vi "Inficon 32 Bit Data.vi"(6 "HHV Manual Mode?":bool, 7 "Gas Type":enum16{"Natural Gas", "Propane Gas"}(ring), 8 "Error In":errorcluster, 9 "Gross Heating Value (Dry) - Manual":sgl, 10 "Inficon Data Input":T3={"Gross Heating Value, Vol (Real, Dry)"=65535.0, "Nitrogen Component Normalized Mole % (Dry)"=8.0, "Methane Component Normalized Mole % (Dry)"=69.0, "Carbon Dioxide Component Normalized Mole % (Dry)"=65535.0, "Ethane Component Normalized Mole % (Dry)"=65.0, "Propane Component Normalized Mole % (Dry)"=8.0, "i-Pentane Component Normalized Mole % (Dry)"=14.0, "i-Butane Component Normalized Mole % (Dry)"=66.0, "n-Butane Component Normalized Mole % (Dry)"=8.0, "n-Pentane Component Normalized Mole % (Dry)"=0.0, "Hexane Component Normalized Mole % (Dry)"=0.0, "Heptane Component Normalized Mole % (Dry)"=0.0, "Gross Wobbe Index, Real(Dry)"=0.0, "Relative Density, Real(Dry)"=40.0, "Propylene Component Normalized Mole % (Dry)"=0.0, "C4 Olefins Component Normalized Mole % (Dry)"=0.0, "Water Component Normalized Mole % (Dry)"=0.0}, 11 "Modbus master in":refnum<class "Modbus Master.lvclass">=refnum) -> (0 "Error Out":errorcluster, 2 "Inficon Data Output":T3, 3 "Modbus master out":refnum<class "Modbus Master.lvclass">, 5 "Text Array":string[][](array[string]))   [LabVIEW 2020]
uses:
  Type Definitions/Inficon Data.ctl
  <vilib>/NI/Modbus Library/API/Master/Modbus Master.lvclass
  <vilib>/NI/Modbus Library/Transmission Data Unit/IP/IP Data Unit.lvclass
  <vilib>/NI/Modbus Library/Master Function Definition/Master Function Definition.lvclass
  <vilib>/NI/Modbus Library/Network Protocol/Network Master/TCP/TCP Master.lvclass
  Type Definitions/Inficon Modbus Addresses.ctl
  Type Definitions/Inficon Modbus Addresses LP.ctl
panel:
  in  "Density LP":T1=126 items=["Gross Heating Value (Dry)"=100, "Ethane"=102, "Propane"=104, "Proplyene"=106, "i-Butane"=108, "n-butane"=110, "C4 Olefins"=112, "Water"=114, "Gross Wobbe Index (Dry)"=124, "Relative Density (Dry)"=126]
  in  "Wobbe LP":T1=124 items=["Gross Heating Value (Dry)"=100, "Ethane"=102, "Propane"=104, "Proplyene"=106, "i-Butane"=108, "n-butane"=110, "C4 Olefins"=112, "Water"=114, "Gross Wobbe Index (Dry)"=124, "Relative Density (Dry)"=126]
  in  "Water":T1=114 items=["Gross Heating Value (Dry)"=100, "Ethane"=102, "Propane"=104, "Proplyene"=106, "i-Butane"=108, "n-butane"=110, "C4 Olefins"=112, "Water"=114, "Gross Wobbe Index (Dry)"=124, "Relative Density (Dry)"=126]
  in  "C4":T1=112 items=["Gross Heating Value (Dry)"=100, "Ethane"=102, "Propane"=104, "Proplyene"=106, "i-Butane"=108, "n-butane"=110, "C4 Olefins"=112, "Water"=114, "Gross Wobbe Index (Dry)"=124, "Relative Density (Dry)"=126]
  in  "n-Butane LP":T1=110 items=["Gross Heating Value (Dry)"=100, "Ethane"=102, "Propane"=104, "Proplyene"=106, "i-Butane"=108, "n-butane"=110, "C4 Olefins"=112, "Water"=114, "Gross Wobbe Index (Dry)"=124, "Relative Density (Dry)"=126]
  in  "i-Butane LP":T1=108 items=["Gross Heating Value (Dry)"=100, "Ethane"=102, "Propane"=104, "Proplyene"=106, "i-Butane"=108, "n-butane"=110, "C4 Olefins"=112, "Water"=114, "Gross Wobbe Index (Dry)"=124, "Relative Density (Dry)"=126]
  in  "Proplyene":T1=106 items=["Gross Heating Value (Dry)"=100, "Ethane"=102, "Propane"=104, "Proplyene"=106, "i-Butane"=108, "n-butane"=110, "C4 Olefins"=112, "Water"=114, "Gross Wobbe Index (Dry)"=124, "Relative Density (Dry)"=126]
  in  "Propane":T1=104 items=["Gross Heating Value (Dry)"=100, "Ethane"=102, "Propane"=104, "Proplyene"=106, "i-Butane"=108, "n-butane"=110, "C4 Olefins"=112, "Water"=114, "Gross Wobbe Index (Dry)"=124, "Relative Density (Dry)"=126]
  in  "Ethane":T1=102 items=["Gross Heating Value (Dry)"=100, "Ethane"=102, "Propane"=104, "Proplyene"=106, "i-Butane"=108, "n-butane"=110, "C4 Olefins"=112, "Water"=114, "Gross Wobbe Index (Dry)"=124, "Relative Density (Dry)"=126]
  in  "HHV LP":T1=100 items=["Gross Heating Value (Dry)"=100, "Ethane"=102, "Propane"=104, "Proplyene"=106, "i-Butane"=108, "n-butane"=110, "C4 Olefins"=112, "Water"=114, "Gross Wobbe Index (Dry)"=124, "Relative Density (Dry)"=126]
  in  "Density NG":T2=126 items=["Gross Heating Value (Dry)"=100, "Nitrogen"=102, "Methane"=104, "CO2"=106, "Ethane"=108, "Propane"=110, "i-Butane"=112, "n-Butane"=114, "i-Pentane"=116, "n-Pentane"=118, "Hexane"=120, "Heptane"=122, "Gross Wobbe Index (Dry)"=124, "Relative Density (Dry)"=126]
  in  "Wobbe NG":T2=124 items=["Gross Heating Value (Dry)"=100, "Nitrogen"=102, "Methane"=104, "CO2"=106, "Ethane"=108, "Propane"=110, "i-Butane"=112, "n-Butane"=114, "i-Pentane"=116, "n-Pentane"=118, "Hexane"=120, "Heptane"=122, "Gross Wobbe Index (Dry)"=124, "Relative Density (Dry)"=126]
  in  "Heptane":T2=122 items=["Gross Heating Value (Dry)"=100, "Nitrogen"=102, "Methane"=104, "CO2"=106, "Ethane"=108, "Propane"=110, "i-Butane"=112, "n-Butane"=114, "i-Pentane"=116, "n-Pentane"=118, "Hexane"=120, "Heptane"=122, "Gross Wobbe Index (Dry)"=124, "Relative Density (Dry)"=126]
  in  "Hexane":T2=120 items=["Gross Heating Value (Dry)"=100, "Nitrogen"=102, "Methane"=104, "CO2"=106, "Ethane"=108, "Propane"=110, "i-Butane"=112, "n-Butane"=114, "i-Pentane"=116, "n-Pentane"=118, "Hexane"=120, "Heptane"=122, "Gross Wobbe Index (Dry)"=124, "Relative Density (Dry)"=126]
  in  "n-Pentane":T2=118 items=["Gross Heating Value (Dry)"=100, "Nitrogen"=102, "Methane"=104, "CO2"=106, "Ethane"=108, "Propane"=110, "i-Butane"=112, "n-Butane"=114, "i-Pentane"=116, "n-Pentane"=118, "Hexane"=120, "Heptane"=122, "Gross Wobbe Index (Dry)"=124, "Relative Density (Dry)"=126]
  in  "i-Pentane":T2=116 items=["Gross Heating Value (Dry)"=100, "Nitrogen"=102, "Methane"=104, "CO2"=106, "Ethane"=108, "Propane"=110, "i-Butane"=112, "n-Butane"=114, "i-Pentane"=116, "n-Pentane"=118, "Hexane"=120, "Heptane"=122, "Gross Wobbe Index (Dry)"=124, "Relative Density (Dry)"=126]
  in  "n-Butane":T2=114 items=["Gross Heating Value (Dry)"=100, "Nitrogen"=102, "Methane"=104, "CO2"=106, "Ethane"=108, "Propane"=110, "i-Butane"=112, "n-Butane"=114, "i-Pentane"=116, "n-Pentane"=118, "Hexane"=120, "Heptane"=122, "Gross Wobbe Index (Dry)"=124, "Relative Density (Dry)"=126]
  in  "i-Butane":T2=112 items=["Gross Heating Value (Dry)"=100, "Nitrogen"=102, "Methane"=104, "CO2"=106, "Ethane"=108, "Propane"=110, "i-Butane"=112, "n-Butane"=114, "i-Pentane"=116, "n-Pentane"=118, "Hexane"=120, "Heptane"=122, "Gross Wobbe Index (Dry)"=124, "Relative Density (Dry)"=126]
  in  "Propane":T2=110 items=["Gross Heating Value (Dry)"=100, "Nitrogen"=102, "Methane"=104, "CO2"=106, "Ethane"=108, "Propane"=110, "i-Butane"=112, "n-Butane"=114, "i-Pentane"=116, "n-Pentane"=118, "Hexane"=120, "Heptane"=122, "Gross Wobbe Index (Dry)"=124, "Relative Density (Dry)"=126]
  in  "Ethane":T2=108 items=["Gross Heating Value (Dry)"=100, "Nitrogen"=102, "Methane"=104, "CO2"=106, "Ethane"=108, "Propane"=110, "i-Butane"=112, "n-Butane"=114, "i-Pentane"=116, "n-Pentane"=118, "Hexane"=120, "Heptane"=122, "Gross Wobbe Index (Dry)"=124, "Relative Density (Dry)"=126]
  in  "CO2":T2=106 items=["Gross Heating Value (Dry)"=100, "Nitrogen"=102, "Methane"=104, "CO2"=106, "Ethane"=108, "Propane"=110, "i-Butane"=112, "n-Butane"=114, "i-Pentane"=116, "n-Pentane"=118, "Hexane"=120, "Heptane"=122, "Gross Wobbe Index (Dry)"=124, "Relative Density (Dry)"=126]
  in  "CH4":T2=104 items=["Gross Heating Value (Dry)"=100, "Nitrogen"=102, "Methane"=104, "CO2"=106, "Ethane"=108, "Propane"=110, "i-Butane"=112, "n-Butane"=114, "i-Pentane"=116, "n-Pentane"=118, "Hexane"=120, "Heptane"=122, "Gross Wobbe Index (Dry)"=124, "Relative Density (Dry)"=126]
  in  "N":T2=102 items=["Gross Heating Value (Dry)"=100, "Nitrogen"=102, "Methane"=104, "CO2"=106, "Ethane"=108, "Propane"=110, "i-Butane"=112, "n-Butane"=114, "i-Pentane"=116, "n-Pentane"=118, "Hexane"=120, "Heptane"=122, "Gross Wobbe Index (Dry)"=124, "Relative Density (Dry)"=126]
  in  "HHV NG":T2=100 items=["Gross Heating Value (Dry)"=100, "Nitrogen"=102, "Methane"=104, "CO2"=106, "Ethane"=108, "Propane"=110, "i-Butane"=112, "n-Butane"=114, "i-Pentane"=116, "n-Pentane"=118, "Hexane"=120, "Heptane"=122, "Gross Wobbe Index (Dry)"=124, "Relative Density (Dry)"=126]
  # "Propane Gas"
  # "Natural Gas"
  # "Natural Gas"
  # "Propane"
  # "Natural Gas"
  # "Propane"
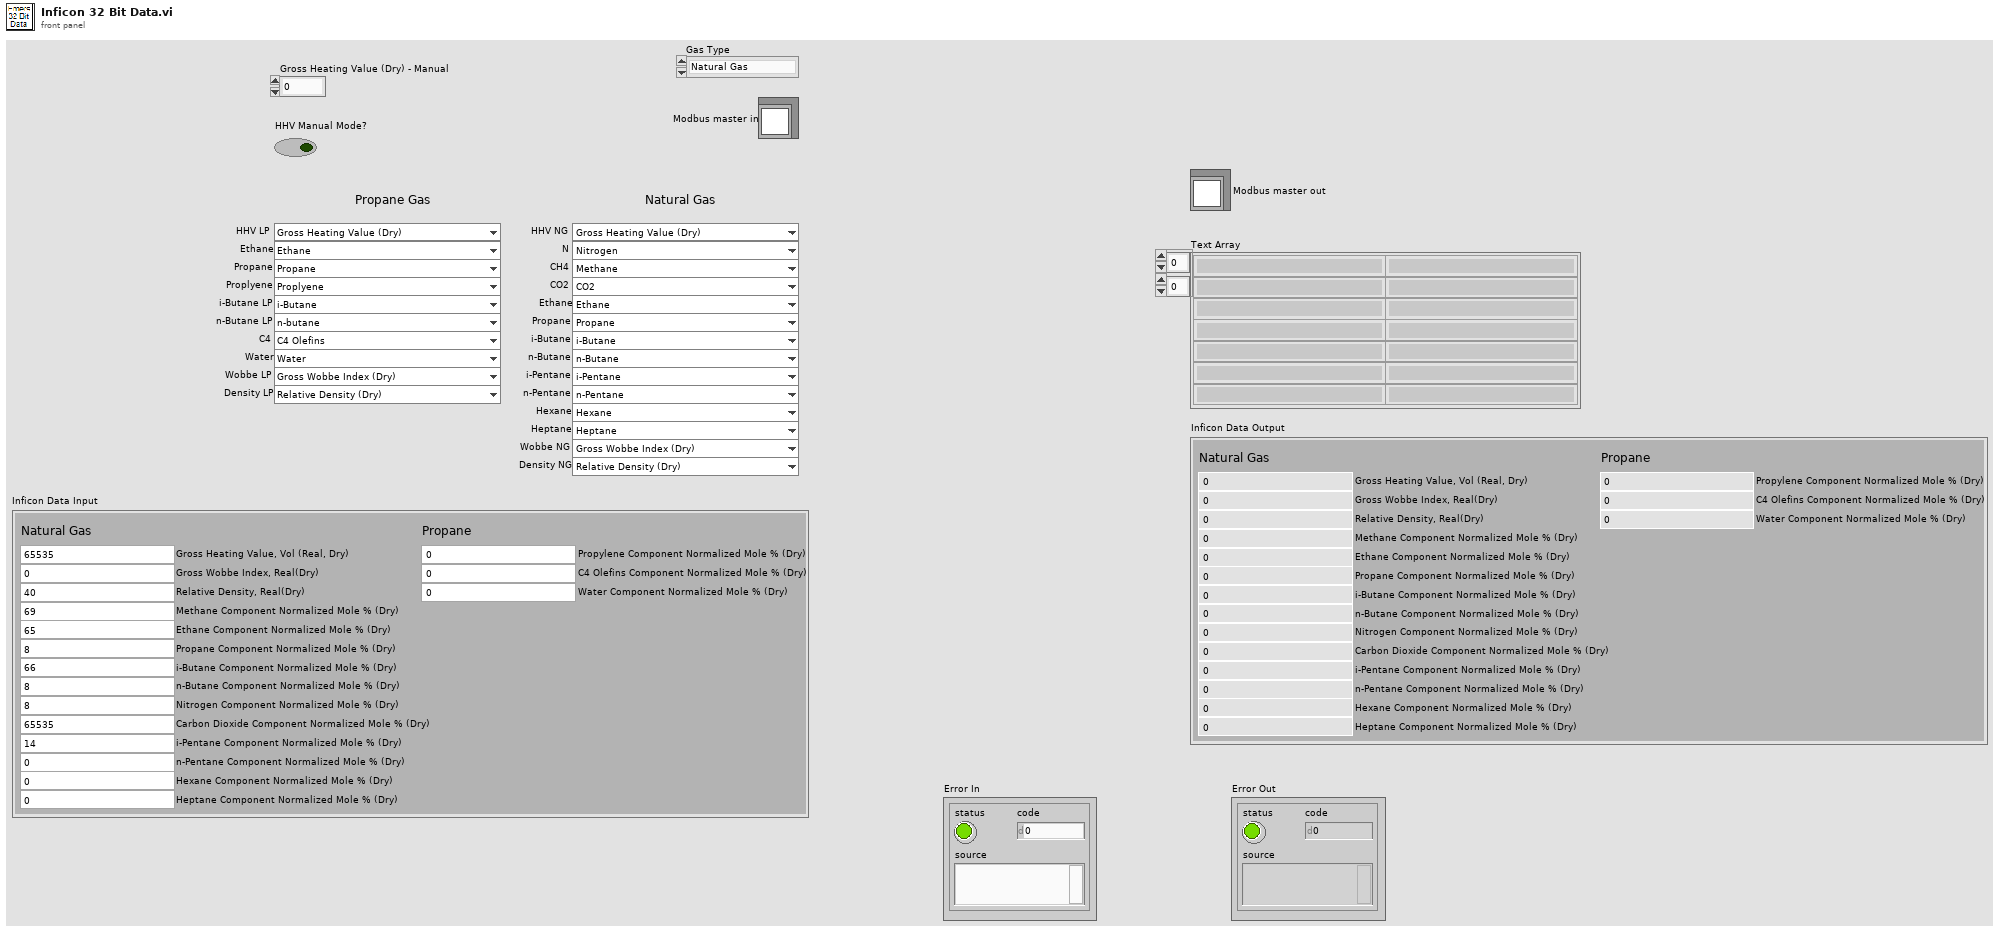
[diagram p1: front panel]
types:
  T1 = typedef "Inficon Modbus Addresses LP.ctl" = u16
  T2 = typedef "Inficon Modbus Addresses.ctl" = u16
  T3 = typedef "Inficon Data.ctl" = cluster{"Gross Heating Value, Vol (Real, Dry)":dbl, "Nitrogen Component Normalized Mole % (Dry)":dbl, "Methane Component Normalized Mole % (Dry)":dbl, "Carbon Dioxide Component Normalized Mole % (Dry)":dbl, "Ethane Component Normalized Mole % (Dry)":dbl, "Propane Component Normalized Mole % (Dry)":dbl, "i-Pentane Component Normalized Mole % (Dry)":dbl, "i-Butane Component Normalized Mole % (Dry)":dbl, "n-Butane Component Normalized Mole % (Dry)":dbl, "n-Pentane Component Normalized Mole % (Dry)":dbl, "Hexane Component Normalized Mole % (Dry)":dbl, "Heptane Component Normalized Mole % (Dry)":dbl, "Gross Wobbe Index, Real(Dry)":dbl, "Relative Density, Real(Dry)":dbl, "Propylene Component Normalized Mole % (Dry)":dbl, "C4 Olefins Component Normalized Mole % (Dry)":dbl, "Water Component Normalized Mole % (Dry)":dbl}
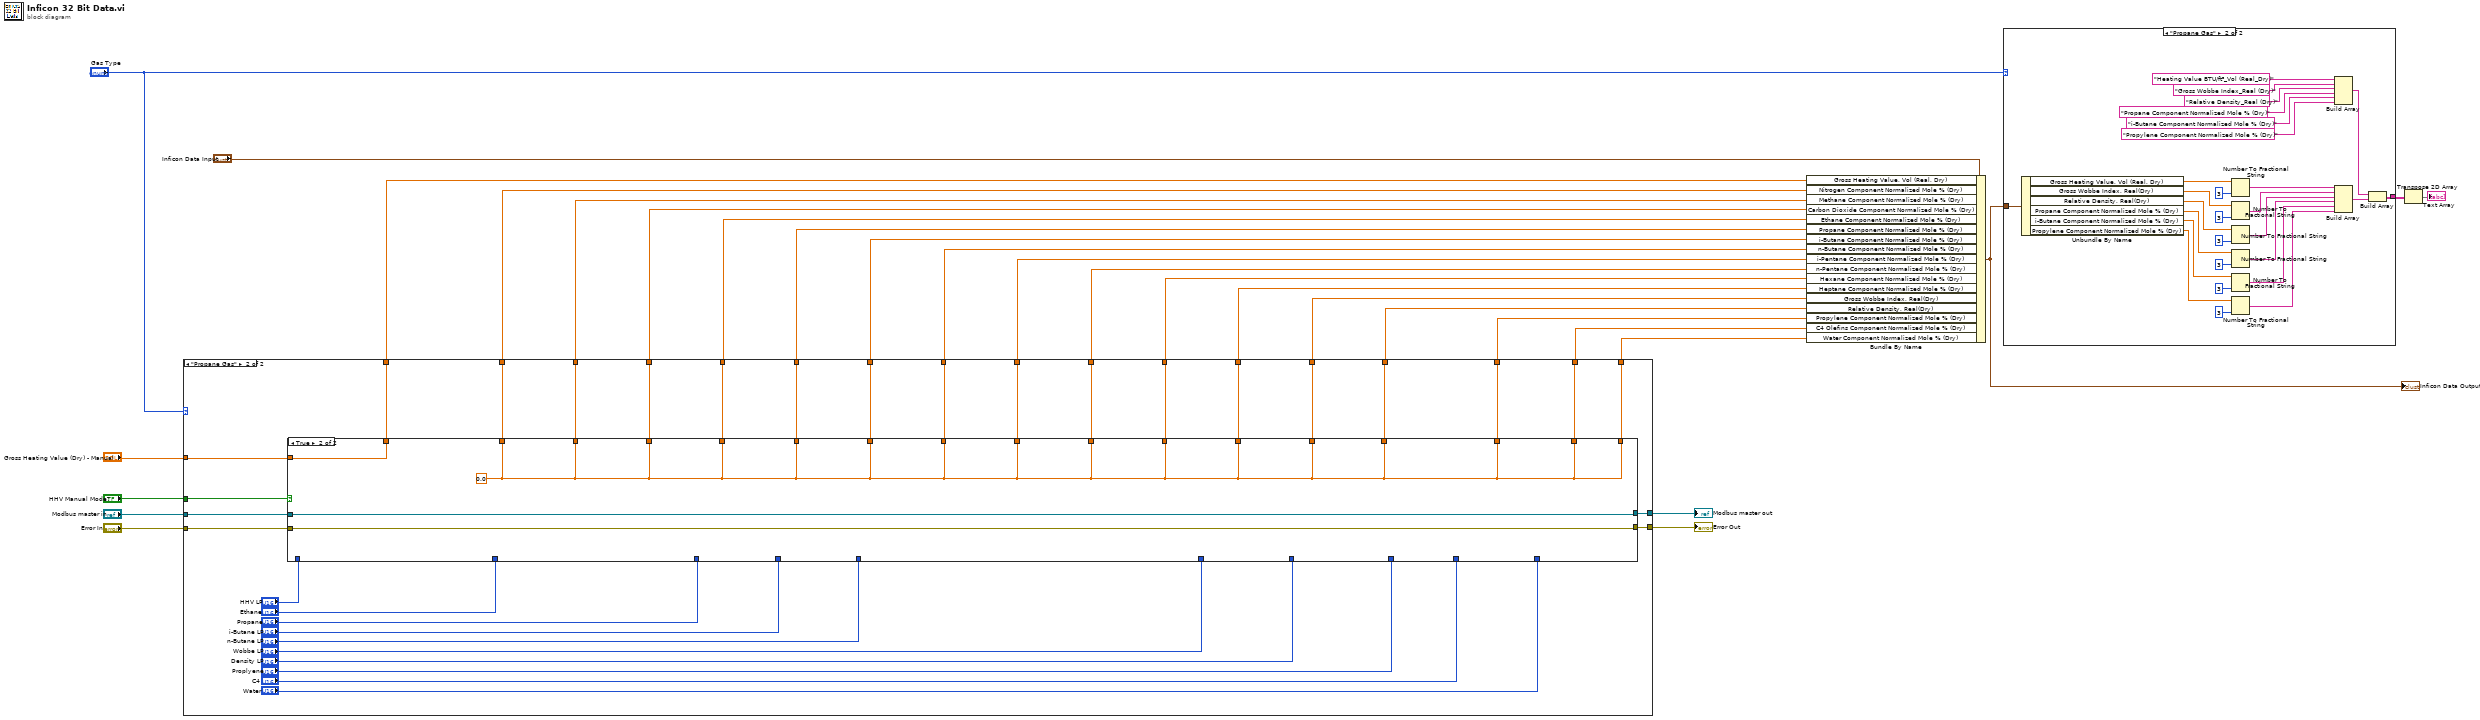
[diagram p0: block diagram]
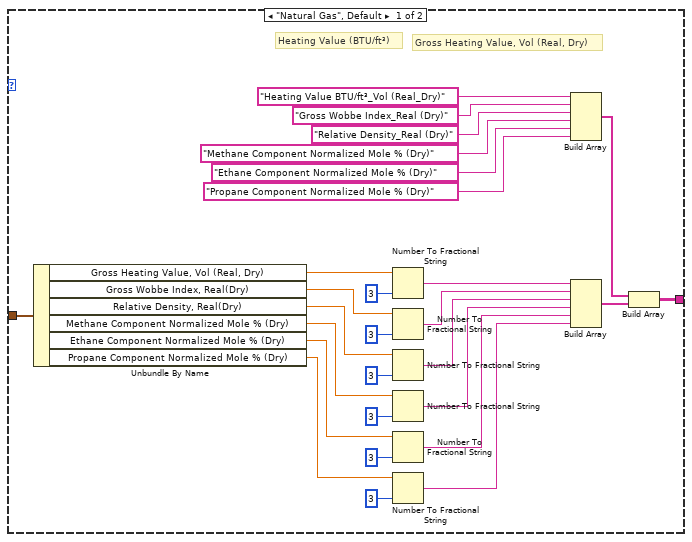
[diagram p2: hidden frame]
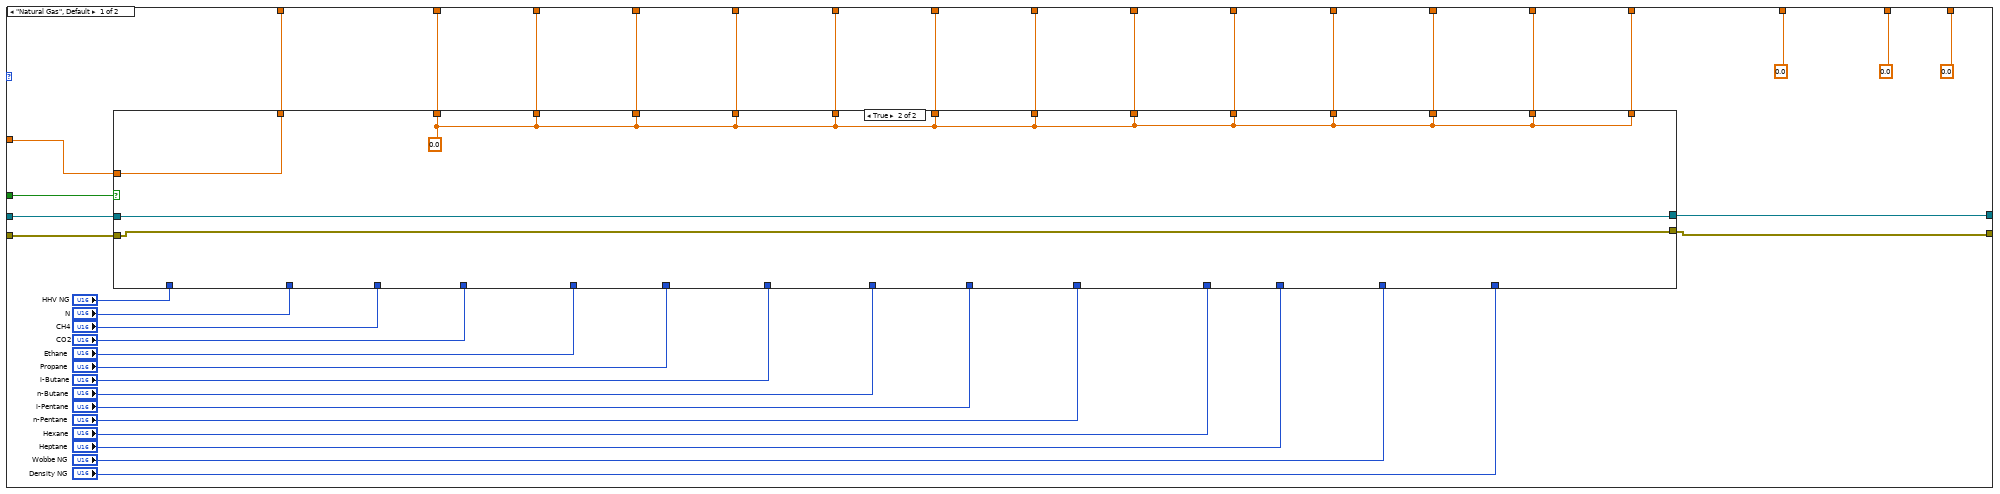
[diagram p3: hidden frame]
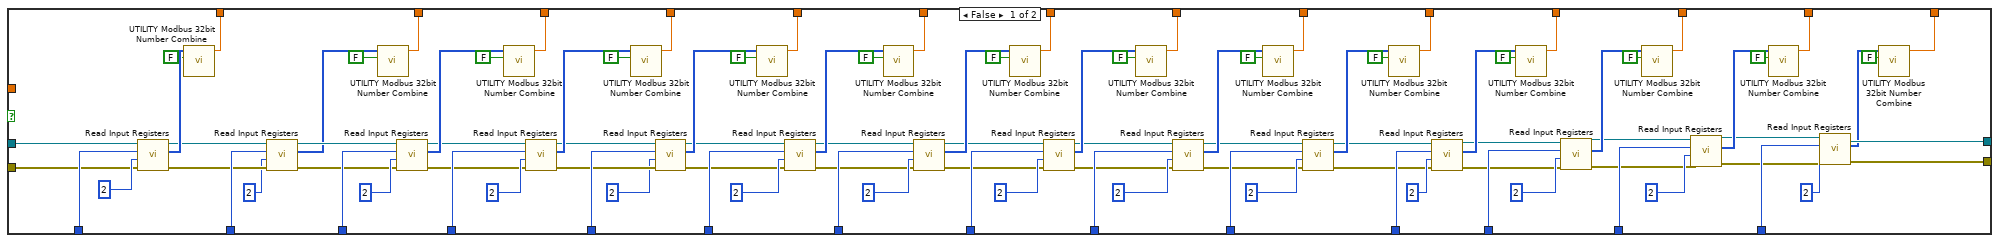
[diagram p4: hidden frame]
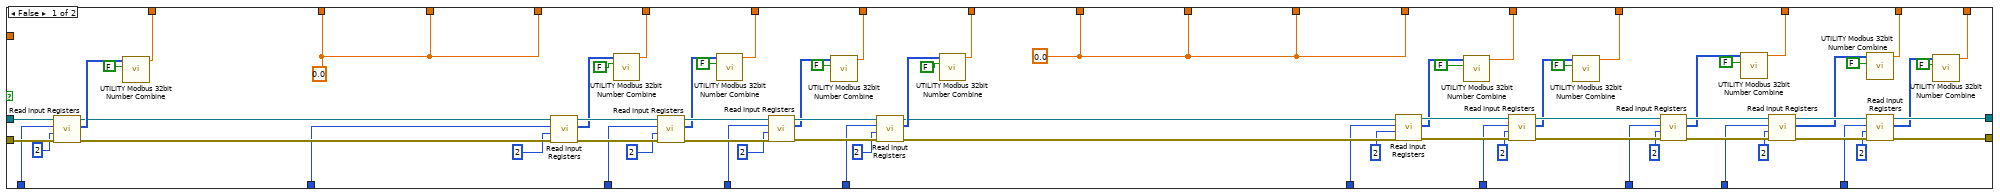
[diagram p5: hidden frame]
diagram:
  n1 = case shown="\"Propane Gas\"" "Gas Type" {
    tunnel: [w65 w194] -> w27
    tunnel: [w64 w193] -> w26
    tunnel: [w63 w202] -> w25
    tunnel: [w62 w201] -> w24
    tunnel: [w61 w192] -> w23
    tunnel: [w60 w199] -> w22
    tunnel: [w59 w191] -> w21
    tunnel: [w58 w190] -> w20
    tunnel: [w57 w189] -> w19
    tunnel: [w56 w200] -> w18
    tunnel: "Modbus master in" -> [w47 w181]
    tunnel: "Error In" -> [w45 w183]
    tunnel: [w43 w171] -> w15
    tunnel: [w42 w170] -> w14
    tunnel: [w41 w198] -> w13
    tunnel: [w40 w197] -> w12
    tunnel: [w39 w188] -> w11
    tunnel: [w38 w187] -> w10
    tunnel: [0.0 ("Propylene Component Normalized Mole % (Dry)") w186] -> w6
    tunnel: [0.0 ("Propylene Component Normalized Mole % (Dry)") w185] -> w5
    tunnel: [0.0 ("Propylene Component Normalized Mole % (Dry)") w184] -> w4
    tunnel: "HHV Manual Mode?" -> [w30 w196]
    tunnel: "Gross Heating Value (Dry) - Manual" -> [w29 w195]
    frame "Natural Gas", Default {
      n2 = case shown="True" w30 {
        tunnel: [w165 w166] -> w65
        tunnel: [w164 w169] -> w64
        tunnel: [w163 w169] -> w63
        tunnel: [w162 w169] -> w62
        tunnel: [w161 w169] -> w61
        tunnel: [w160 w169] -> w60
        tunnel: [w159 w169] -> w59
        tunnel: [w158 w169] -> w58
        tunnel: [w157 w169] -> w57
        tunnel: [w156 w169] -> w56
        tunnel: "CH4" -> [w155 _]
        tunnel: "CO2" -> [w154 _]
        tunnel: "Ethane" -> [w153 _]
        tunnel: "Propane" -> [w152 _]
        tunnel: "i-Butane" -> [w151 _]
        tunnel: "n-Butane" -> [w150 _]
        tunnel: "i-Pentane" -> [w149 _]
        tunnel: "n-Pentane" -> [w148 _]
        tunnel: w47 -> [w147 w167]
        tunnel: "HHV NG" -> [w146 _]
        tunnel: w45 -> [w143 w168]
        tunnel: "N" -> [w140 _]
        tunnel: [w138 w168] -> w43
        tunnel: [w137 w167] -> w42
        tunnel: [w136 w169] -> w41
        tunnel: [w135 w169] -> w40
        tunnel: [w134 w169] -> w39
        tunnel: [w133 w169] -> w38
        tunnel: "Hexane" -> [w132 _]
        tunnel: "Heptane" -> [w131 _]
        tunnel: "Wobbe NG" -> [w130 _]
        tunnel: "Density NG" -> [w129 _]
        tunnel: w29 -> [_ w166]
        frame False {
          n3 = call-dynamic "Read Input Registers.vi"("error in"=w143, "number of inputs"=u16 2 ("Quantity"), "starting address"=w146, "Modbus master in"=w147) -> ("error out"=w139:errorcluster, "register values"=w144:u16[], "Modbus master out"=w141:refnum<class "Modbus Master.lvclass">)  [unwired: 5 in]
          n4 = call "UTILITY Modbus 32bit Number Combine.vi"("Swap Words"=FALSE, "Holding Registers"=w144) -> ("Data"=w165:sgl)  [unwired: 8 in, 1 out]
          n5 = call-dynamic "Read Input Registers.vi"("error in"=w139, "number of inputs"=u16 2 ("Quantity"), "starting address"=w140, "Modbus master in"=w141) -> ("error out"=w94:errorcluster, "register values"=w95:u16[], "Modbus master out"=w96:refnum<class "Modbus Master.lvclass">)  [unwired: 5 in]
          n6 = call "UTILITY Modbus 32bit Number Combine.vi"("Swap Words"=FALSE, "Holding Registers"=w95) -> ("Data"=w164:sgl)  [unwired: 8 in, 1 out]
          n7 = call-dynamic "Read Input Registers.vi"("error in"=w94, "number of inputs"=u16 2 ("Quantity"), "starting address"=w155, "Modbus master in"=w96) -> ("error out"=w121:errorcluster, "register values"=w127:u16[], "Modbus master out"=w123:refnum<class "Modbus Master.lvclass">)  [unwired: 5 in]
          n8 = call "UTILITY Modbus 32bit Number Combine.vi"("Swap Words"=FALSE, "Holding Registers"=w127) -> ("Data"=w163:sgl)  [unwired: 8 in, 1 out]
          n9 = call-dynamic "Read Input Registers.vi"("error in"=w121, "number of inputs"=u16 2 ("Quantity"), "starting address"=w154, "Modbus master in"=w123) -> ("error out"=w120:errorcluster, "register values"=w126:u16[], "Modbus master out"=w122:refnum<class "Modbus Master.lvclass">)  [unwired: 5 in]
          n10 = call "UTILITY Modbus 32bit Number Combine.vi"("Swap Words"=FALSE, "Holding Registers"=w126) -> ("Data"=w162:sgl)  [unwired: 8 in, 1 out]
          n11 = call-dynamic "Read Input Registers.vi"("error in"=w120, "number of inputs"=u16 2 ("Quantity"), "starting address"=w153, "Modbus master in"=w122) -> ("error out"=w109:errorcluster, "register values"=w124:u16[], "Modbus master out"=w104:refnum<class "Modbus Master.lvclass">)  [unwired: 5 in]
          n12 = call "UTILITY Modbus 32bit Number Combine.vi"("Swap Words"=FALSE, "Holding Registers"=w124) -> ("Data"=w161:sgl)  [unwired: 8 in, 1 out]
          n13 = call-dynamic "Read Input Registers.vi"("error in"=w109, "number of inputs"=u16 2 ("Quantity"), "starting address"=w152, "Modbus master in"=w104) -> ("error out"=w108:errorcluster, "register values"=w119:u16[], "Modbus master out"=w103:refnum<class "Modbus Master.lvclass">)  [unwired: 5 in]
          n14 = call "UTILITY Modbus 32bit Number Combine.vi"("Swap Words"=FALSE, "Holding Registers"=w119) -> ("Data"=w159:sgl)  [unwired: 8 in, 1 out]
          n15 = call-dynamic "Read Input Registers.vi"("error in"=w108, "number of inputs"=u16 2 ("Quantity"), "starting address"=w151, "Modbus master in"=w103) -> ("error out"=w107:errorcluster, "register values"=w116:u16[], "Modbus master out"=w102:refnum<class "Modbus Master.lvclass">)  [unwired: 5 in]
          n16 = call "UTILITY Modbus 32bit Number Combine.vi"("Swap Words"=FALSE, "Holding Registers"=w116) -> ("Data"=w158:sgl)  [unwired: 8 in, 1 out]
          n17 = call-dynamic "Read Input Registers.vi"("error in"=w107, "number of inputs"=u16 2 ("Quantity"), "starting address"=w150, "Modbus master in"=w102) -> ("error out"=w106:errorcluster, "register values"=w115:u16[], "Modbus master out"=w101:refnum<class "Modbus Master.lvclass">)  [unwired: 5 in]
          n18 = call "UTILITY Modbus 32bit Number Combine.vi"("Swap Words"=FALSE, "Holding Registers"=w115) -> ("Data"=w157:sgl)  [unwired: 8 in, 1 out]
          n19 = call-dynamic "Read Input Registers.vi"("error in"=w106, "number of inputs"=u16 2 ("Quantity"), "starting address"=w149, "Modbus master in"=w101) -> ("error out"=w105:errorcluster, "register values"=w112:u16[], "Modbus master out"=w100:refnum<class "Modbus Master.lvclass">)  [unwired: 5 in]
          n20 = call "UTILITY Modbus 32bit Number Combine.vi"("Swap Words"=FALSE, "Holding Registers"=w112) -> ("Data"=w156:sgl)  [unwired: 8 in, 1 out]
          n21 = call-dynamic "Read Input Registers.vi"("error in"=w105, "number of inputs"=u16 2 ("Quantity"), "starting address"=w148, "Modbus master in"=w100) -> ("error out"=w74:errorcluster, "register values"=w111:u16[], "Modbus master out"=w67:refnum<class "Modbus Master.lvclass">)  [unwired: 5 in]
          n22 = call "UTILITY Modbus 32bit Number Combine.vi"("Swap Words"=FALSE, "Holding Registers"=w111) -> ("Data"=w160:sgl)  [unwired: 8 in, 1 out]
          n23 = call-dynamic "Read Input Registers.vi"("error in"=w74, "number of inputs"=u16 2 ("Quantity"), "starting address"=w132, "Modbus master in"=w67) -> ("error out"=w73:errorcluster, "register values"=w83:u16[], "Modbus master out"=w68:refnum<class "Modbus Master.lvclass">)  [unwired: 5 in]
          n24 = call "UTILITY Modbus 32bit Number Combine.vi"("Swap Words"=FALSE, "Holding Registers"=w83) -> ("Data"=w136:sgl)  [unwired: 8 in, 1 out]
          n25 = call-dynamic "Read Input Registers.vi"("error in"=w73, "number of inputs"=u16 2 ("Quantity"), "starting address"=w131, "Modbus master in"=w68) -> ("error out"=w72:errorcluster, "register values"=w82:u16[], "Modbus master out"=w69:refnum<class "Modbus Master.lvclass">)  [unwired: 5 in]
          n26 = call "UTILITY Modbus 32bit Number Combine.vi"("Swap Words"=FALSE, "Holding Registers"=w82) -> ("Data"=w135:sgl)  [unwired: 8 in, 1 out]
          n27 = call-dynamic "Read Input Registers.vi"("error in"=w72, "number of inputs"=u16 2 ("Quantity"), "starting address"=w130, "Modbus master in"=w69) -> ("error out"=w71:errorcluster, "register values"=w77:u16[], "Modbus master out"=w70:refnum<class "Modbus Master.lvclass">)  [unwired: 5 in]
          n28 = call "UTILITY Modbus 32bit Number Combine.vi"("Swap Words"=FALSE, "Holding Registers"=w77) -> ("Data"=w134:sgl)  [unwired: 8 in, 1 out]
          n29 = call-dynamic "Read Input Registers.vi"("error in"=w71, "number of inputs"=u16 2 ("Quantity"), "starting address"=w129, "Modbus master in"=w70) -> ("error out"=w138:errorcluster, "register values"=w66:u16[], "Modbus master out"=w137:refnum<class "Modbus Master.lvclass">)  [unwired: 5 in]
          n30 = call "UTILITY Modbus 32bit Number Combine.vi"("Swap Words"=FALSE, "Holding Registers"=w66) -> ("Data"=w133:sgl)  [unwired: 8 in, 1 out]
        }
        frame True {
          w169 = sgl 0.0 ("Data")
        }
      }
    }
    frame "Propane Gas" {
      n31 = case shown="True" w196 {
        tunnel: [w275 w280] -> w202
        tunnel: [w275 w280] -> w201
        tunnel: [w276 w280] -> w200
        tunnel: [w276 w280] -> w199
        tunnel: [w276 w280] -> w198
        tunnel: [w276 w280] -> w197
        tunnel: w195 -> [_ w279]
        tunnel: [w203 w279] -> w194
        tunnel: [w275 w280] -> w193
        tunnel: [w272 w280] -> w192
        tunnel: [w266 w280] -> w191
        tunnel: [w267 w280] -> w190
        tunnel: [w268 w280] -> w189
        tunnel: [w209 w280] -> w188
        tunnel: [w210 w280] -> w187
        tunnel: [w211 w280] -> w186
        tunnel: [w212 w280] -> w185
        tunnel: [w213 w280] -> w184
        tunnel: w183 -> [w265 w278]
        tunnel: "HHV LP" -> [w263 _]
        tunnel: w181 -> [w262 w277]
        tunnel: "n-Butane LP" -> [w253 _]
        tunnel: "i-Butane LP" -> [w251 _]
        tunnel: "Propane" -> [w249 _]
        tunnel: "Ethane" -> [w246 _]
        tunnel: "Water" -> [w231 _]
        tunnel: "C4" -> [w228 _]
        tunnel: "Proplyene" -> [w225 _]
        tunnel: "Density LP" -> [w221 _]
        tunnel: "Wobbe LP" -> [w217 _]
        tunnel: [w215 w278] -> w171
        tunnel: [w214 w277] -> w170
        frame False {
          w275 = sgl 0.0 ("Data")
          w276 = sgl 0.0 ("Data")
          n32 = call-dynamic "Read Input Registers.vi"("error in"=w265, "number of inputs"=u16 2 ("Quantity"), "starting address"=w263, "Modbus master in"=w262) -> ("error out"=w248:errorcluster, "register values"=w261:u16[], "Modbus master out"=w245:refnum<class "Modbus Master.lvclass">)  [unwired: 5 in]
          n33 = call "UTILITY Modbus 32bit Number Combine.vi"("Swap Words"=FALSE, "Holding Registers"=w261) -> ("Data"=w203:sgl)  [unwired: 8 in, 1 out]
          n34 = call-dynamic "Read Input Registers.vi"("error in"=w248, "number of inputs"=u16 2 ("Quantity"), "starting address"=w246, "Modbus master in"=w245) -> ("error out"=w255:errorcluster, "register values"=w242:u16[], "Modbus master out"=w258:refnum<class "Modbus Master.lvclass">)  [unwired: 5 in]
          n35 = call "UTILITY Modbus 32bit Number Combine.vi"("Swap Words"=FALSE, "Holding Registers"=w242) -> ("Data"=w272:sgl)  [unwired: 8 in, 1 out]
          n36 = call-dynamic "Read Input Registers.vi"("error in"=w255, "number of inputs"=u16 2 ("Quantity"), "starting address"=w249, "Modbus master in"=w258) -> ("error out"=w256:errorcluster, "register values"=w243:u16[], "Modbus master out"=w257:refnum<class "Modbus Master.lvclass">)  [unwired: 5 in]
          n37 = call "UTILITY Modbus 32bit Number Combine.vi"("Swap Words"=FALSE, "Holding Registers"=w243) -> ("Data"=w266:sgl)  [unwired: 8 in, 1 out]
          n38 = call-dynamic "Read Input Registers.vi"("error in"=w256, "number of inputs"=u16 2 ("Quantity"), "starting address"=w251, "Modbus master in"=w257) -> ("error out"=w259:errorcluster, "register values"=w241:u16[], "Modbus master out"=w260:refnum<class "Modbus Master.lvclass">)  [unwired: 5 in]
          n39 = call "UTILITY Modbus 32bit Number Combine.vi"("Swap Words"=FALSE, "Holding Registers"=w241) -> ("Data"=w267:sgl)  [unwired: 8 in, 1 out]
          n40 = call-dynamic "Read Input Registers.vi"("error in"=w259, "number of inputs"=u16 2 ("Quantity"), "starting address"=w253, "Modbus master in"=w260) -> ("error out"=w219:errorcluster, "register values"=w244:u16[], "Modbus master out"=w216:refnum<class "Modbus Master.lvclass">)  [unwired: 5 in]
          n41 = call "UTILITY Modbus 32bit Number Combine.vi"("Swap Words"=FALSE, "Holding Registers"=w244) -> ("Data"=w268:sgl)  [unwired: 8 in, 1 out]
          n42 = call-dynamic "Read Input Registers.vi"("error in"=w219, "number of inputs"=u16 2 ("Quantity"), "starting address"=w217, "Modbus master in"=w216) -> ("error out"=w233:errorcluster, "register values"=w207:u16[], "Modbus master out"=w234:refnum<class "Modbus Master.lvclass">)  [unwired: 5 in]
          n43 = call "UTILITY Modbus 32bit Number Combine.vi"("Swap Words"=FALSE, "Holding Registers"=w207) -> ("Data"=w209:sgl)  [unwired: 8 in, 1 out]
          n44 = call-dynamic "Read Input Registers.vi"("error in"=w233, "number of inputs"=u16 2 ("Quantity"), "starting address"=w221, "Modbus master in"=w234) -> ("error out"=w235:errorcluster, "register values"=w208:u16[], "Modbus master out"=w236:refnum<class "Modbus Master.lvclass">)  [unwired: 5 in]
          n45 = call "UTILITY Modbus 32bit Number Combine.vi"("Swap Words"=FALSE, "Holding Registers"=w208) -> ("Data"=w210:sgl)  [unwired: 8 in, 1 out]
          n46 = call-dynamic "Read Input Registers.vi"("error in"=w235, "number of inputs"=u16 2 ("Quantity"), "starting address"=w225, "Modbus master in"=w236) -> ("error out"=w238:errorcluster, "register values"=w206:u16[], "Modbus master out"=w237:refnum<class "Modbus Master.lvclass">)  [unwired: 5 in]
          n47 = call "UTILITY Modbus 32bit Number Combine.vi"("Swap Words"=FALSE, "Holding Registers"=w206) -> ("Data"=w211:sgl)  [unwired: 8 in, 1 out]
          n48 = call-dynamic "Read Input Registers.vi"("error in"=w238, "number of inputs"=u16 2 ("Quantity"), "starting address"=w228, "Modbus master in"=w237) -> ("error out"=w239:errorcluster, "register values"=w205:u16[], "Modbus master out"=w240:refnum<class "Modbus Master.lvclass">)  [unwired: 5 in]
          n49 = call "UTILITY Modbus 32bit Number Combine.vi"("Swap Words"=FALSE, "Holding Registers"=w205) -> ("Data"=w212:sgl)  [unwired: 8 in, 1 out]
          n50 = call-dynamic "Read Input Registers.vi"("error in"=w239, "number of inputs"=u16 2 ("Quantity"), "starting address"=w231, "Modbus master in"=w240) -> ("error out"=w215:errorcluster, "register values"=w204:u16[], "Modbus master out"=w214:refnum<class "Modbus Master.lvclass">)  [unwired: 5 in]
          n51 = call "UTILITY Modbus 32bit Number Combine.vi"("Swap Words"=FALSE, "Holding Registers"=w204) -> ("Data"=w213:sgl)  [unwired: 8 in, 1 out]
        }
        frame True {
          w280 = sgl 0.0 ("Data")
        }
      }
    }
  }
  "Error Out" <- w15
  "Modbus master out" <- w14
  n52 = Bundle By Name(cluster="Inficon Data Input", "Gross Heating Value, Vol (Real, Dry)"=w27, "Nitrogen Component Normalized Mole % (Dry)"=w26, "Methane Component Normalized Mole % (Dry)"=w25, "Carbon Dioxide Component Normalized Mole % (Dry)"=w24, "Ethane Component Normalized Mole % (Dry)"=w23, "Propane Component Normalized Mole % (Dry)"=w21, "i-Butane Component Normalized Mole % (Dry)"=w20, "n-Butane Component Normalized Mole % (Dry)"=w19, "i-Pentane Component Normalized Mole % (Dry)"=w18, "n-Pentane Component Normalized Mole % (Dry)"=w22, "Hexane Component Normalized Mole % (Dry)"=w13, "Heptane Component Normalized Mole % (Dry)"=w12, "Gross Wobbe Index, Real(Dry)"=w11, "Relative Density, Real(Dry)"=w10, "Propylene Component Normalized Mole % (Dry)"=w6, "C4 Olefins Component Normalized Mole % (Dry)"=w5, "Water Component Normalized Mole % (Dry)"=w4) -> (w9:T3)
  "Inficon Data Output" <- w9
  n53 = case shown="\"Propane Gas\"" "Gas Type" {
    tunnel: w9 -> [w308 w309]
    tunnel: [w301 w310] -> w8
    frame "Natural Gas", Default {
      # "Gross Heating Value, Vol (Real, Dry)"
      # "Heating Value (BTU/ft³)"
      n54 = Unbundle By Name(w308) -> ("Gross Heating Value, Vol (Real, Dry)"=w307:dbl, "Gross Wobbe Index, Real(Dry)"=w295:dbl, "Relative Density, Real(Dry)"=w294:dbl, "Methane Component Normalized Mole % (Dry)"=w293:dbl, "Ethane Component Normalized Mole % (Dry)"=w292:dbl, "Propane Component Normalized Mole % (Dry)"=w291:dbl)
      n55 = Number To Fractional String(number=w307, precision (6)=i16 3) -> (F-format string=w304:string)  [unwired: 2 in]
      n56 = Number To Fractional String(number=w295, precision (6)=i16 3) -> (F-format string=w290:string)  [unwired: 2 in]
      n57 = Number To Fractional String(number=w294, precision (6)=i16 3) -> (F-format string=w289:string)  [unwired: 2 in]
      n58 = Number To Fractional String(number=w293, precision (6)=i16 3) -> (F-format string=w288:string)  [unwired: 2 in]
      n59 = Number To Fractional String(number=w292, precision (6)=i16 3) -> (F-format string=w287:string)  [unwired: 2 in]
      n60 = Number To Fractional String(number=w291, precision (6)=i16 3) -> (F-format string=w286:string)  [unwired: 2 in]
      n61 = Build Array("Heating Value BTU/ft³_Vol (Real_Dry)", "Gross Wobbe Index_Real (Dry)", "Relative Density_Real (Dry)", "Methane Component Normalized Mole % (Dry)", "Ethane Component Normalized Mole % (Dry)", "Propane Component Normalized Mole % (Dry)") -> (w303:string[])
      n62 = Build Array(w304, w290, w289, w288, w287, w286) -> (w302:string[])
      n63 = Build Array(w303, w302) -> (w301:string[][])
    }
    frame "Propane Gas" {
      n64 = Unbundle By Name(w309) -> ("Gross Heating Value, Vol (Real, Dry)"=w336:dbl, "Gross Wobbe Index, Real(Dry)"=w332:dbl, "Relative Density, Real(Dry)"=w331:dbl, "Propane Component Normalized Mole % (Dry)"=w330:dbl, "i-Butane Component Normalized Mole % (Dry)"=w329:dbl, "Propylene Component Normalized Mole % (Dry)"=w328:dbl)
      n65 = Number To Fractional String(number=w336, precision (6)=i16 3) -> (F-format string=w335:string)  [unwired: 2 in]
      n66 = Number To Fractional String(number=w332, precision (6)=i16 3) -> (F-format string=w327:string)  [unwired: 2 in]
      n67 = Number To Fractional String(number=w331, precision (6)=i16 3) -> (F-format string=w326:string)  [unwired: 2 in]
      n68 = Number To Fractional String(number=w330, precision (6)=i16 3) -> (F-format string=w325:string)  [unwired: 2 in]
      n69 = Number To Fractional String(number=w329, precision (6)=i16 3) -> (F-format string=w324:string)  [unwired: 2 in]
      n70 = Number To Fractional String(number=w328, precision (6)=i16 3) -> (F-format string=w323:string)  [unwired: 2 in]
      n71 = Build Array("Heating Value BTU/ft³_Vol (Real_Dry)", "Gross Wobbe Index_Real (Dry)", "Relative Density_Real (Dry)", "Propane Component Normalized Mole % (Dry)", "i-Butane Component Normalized Mole % (Dry)", "Propylene Component Normalized Mole % (Dry)") -> (w334:string[])
      n72 = Build Array(w335, w327, w326, w325, w324, w323) -> (w333:string[])
      n73 = Build Array(w334, w333) -> (w310:string[][])
    }
  }
  n74 = Transpose 2D Array(2D array=w8) -> (transposed array=→"Text Array":string[][])
